vi "VibSystem2Signals.vi"(8 "sampling info":cluster{"Fs":dbl, "#s":dbl}={"Fs"=10000.0, "#s"=10000.0} {"Fs" format="%.2p"}, 10 "Frequency":dbl, 11 "Constant Amplitudes?":bool) -> (3 "Signals":waveform(dbl)[](array[waveform]))   [LabVIEW 2017]
uses:
  <vilib>/measure/NI_MABase.lvlib
panel:
  out "Waveform Graph":waveform(dbl)[](graph)
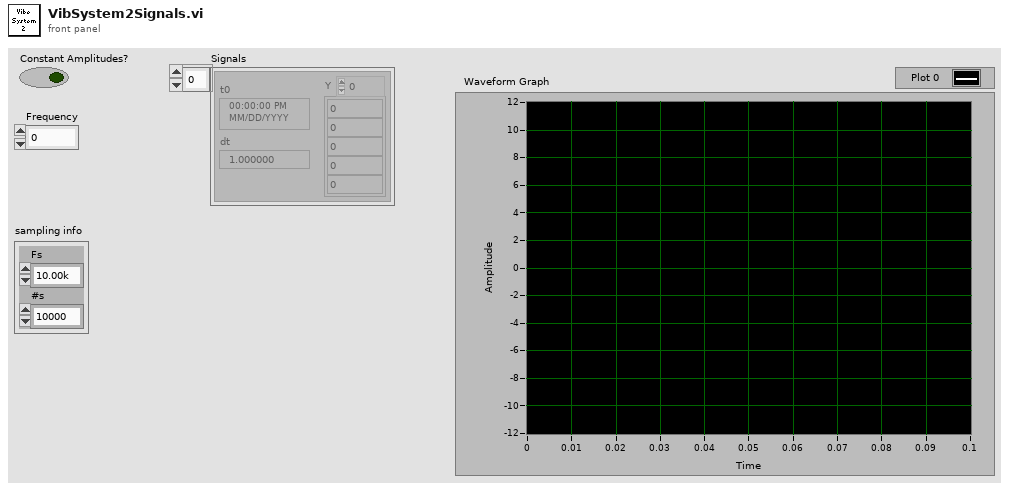
[diagram p1: front panel]
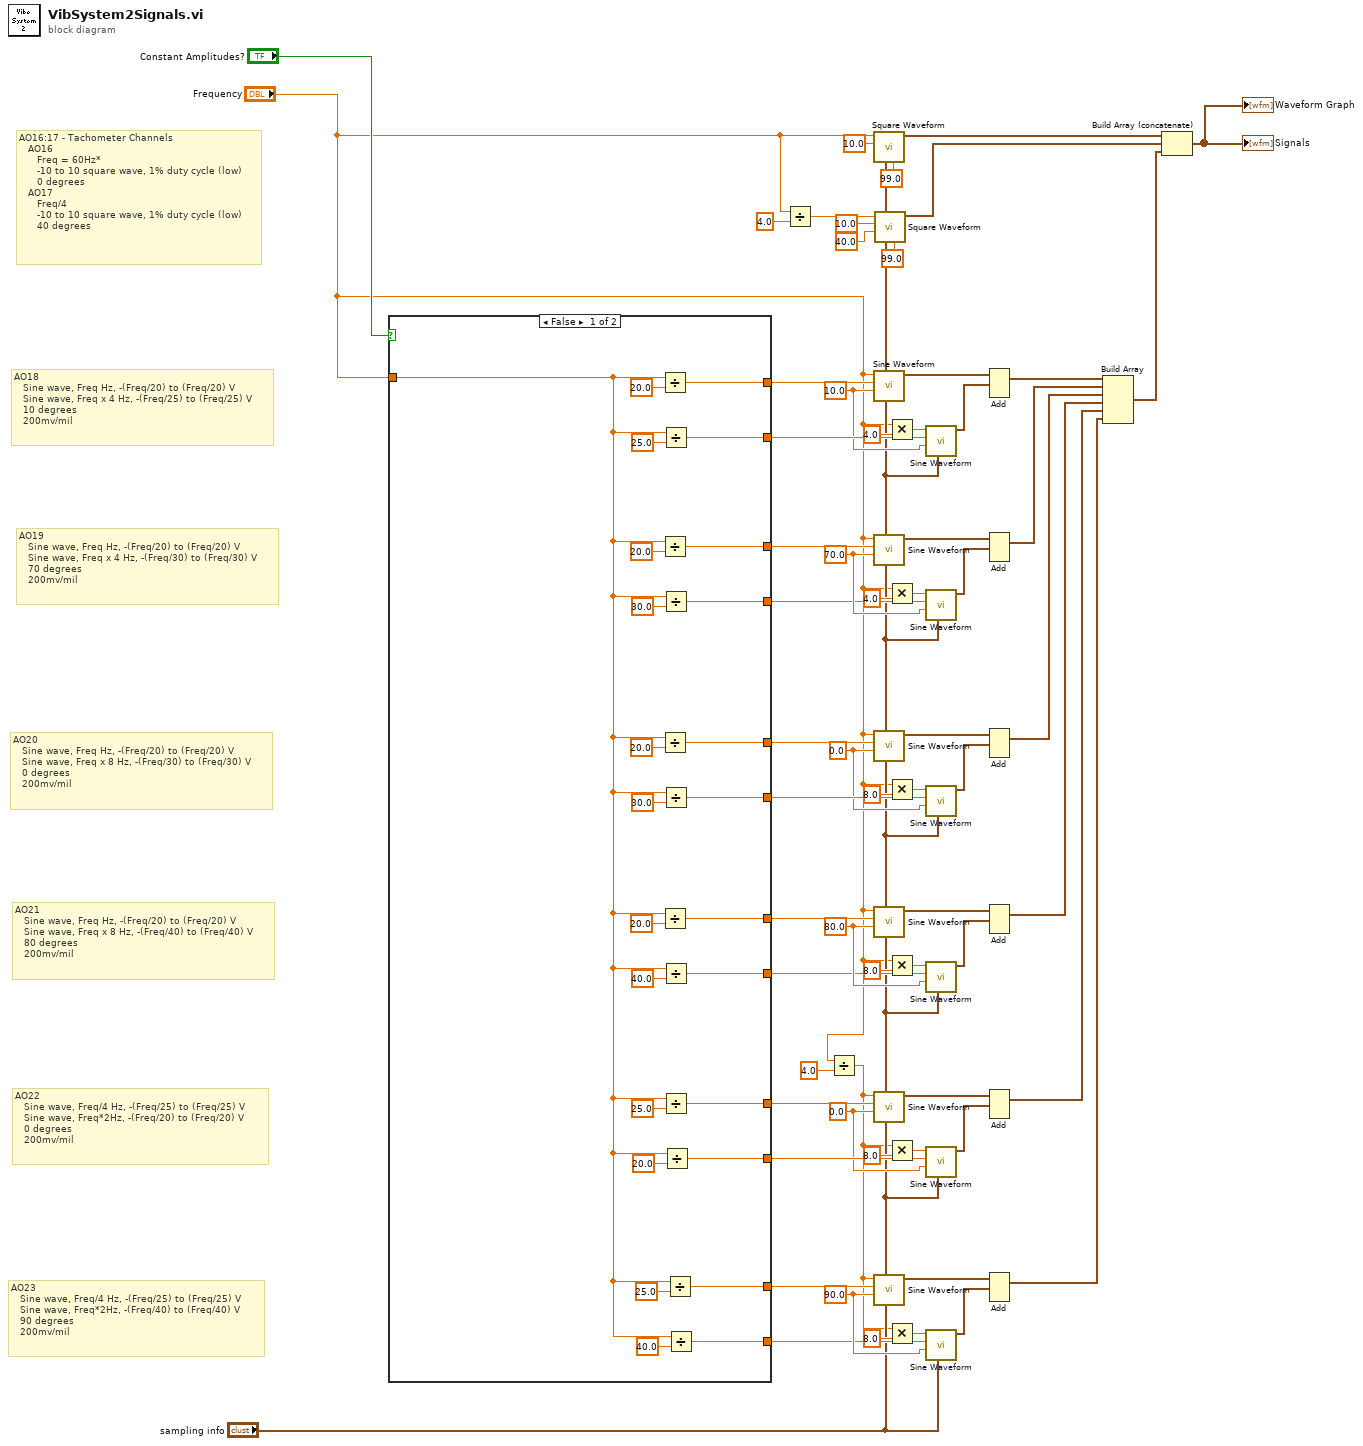
[diagram p0: block diagram]
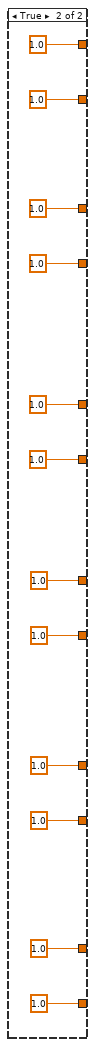
[diagram p2: hidden frame]
diagram:
  w9 = 90.0 ("phase")
  w18 = 0.0 ("phase")
  w24 = 80.0 ("phase")
  w34 = 0.0 ("phase")
  w40 = 70.0 ("phase")
  w60 = 10.0 ("phase")
  # "AO23\n   Sine wave, Freq/4 Hz, -(Freq/25) to (Freq/25) V\n   Sine wave, Freq*2Hz, -(Freq/40) to (Freq/40) V\n   90 degrees\n   200mv/mil"
  # "AO22\n   Sine wave, Freq/4 Hz, -(Freq/25) to (Freq/25) V\n   Sine wave, Freq*2Hz, -(Freq/20) to (Freq/20) V\n   0 degrees\n   200mv/mil"
  # "AO21\n   Sine wave, Freq Hz, -(Freq/20) to (Freq/20) V\n   Sine wave, Freq x 8 Hz, -(Freq/40) to (Freq/40) V\n   80 degrees\n   200mv/mil"
  # "AO19\n   Sine wave, Freq Hz, -(Freq/20) to (Freq/20) V\n   Sine wave, Freq x 4 Hz, -(Freq/30) to (Freq/30) V\n   70 degrees\n   200mv/mil"
  # "AO20\n   Sine wave, Freq Hz, -(Freq/20) to (Freq/20) V\n   Sine wave, Freq x 8 Hz, -(Freq/30) to (Freq/30) V\n   0 degrees\n   200mv/mil"
  # "AO18\n   Sine wave, Freq Hz, -(Freq/20) to (Freq/20) V\n   Sine wave, Freq x 4 Hz, -(Freq/25) to (Freq/25) V\n   10 degrees\n   200mv/mil"
  # "AO16:17 - Tachometer Channels\n   AO16\n      Freq = 60Hz*\n      -10 to 10 square wave, 1% duty cycle (low)\n      0 degrees\n   AO17\n      Freq/4\n      -10 to 10 square wave, 1% duty cycle (low)\n      40 degrees"
  n1 = case shown="False" "Constant Amplitudes?" {
    tunnel: [w87 1.0] -> w62
    tunnel: [w86 1.0] -> w63
    tunnel: "Frequency" -> [w69 _]
    tunnel: [w84 1.0] -> w39
    tunnel: [w85 1.0] -> w38
    tunnel: [w79 1.0] -> w35
    tunnel: [w78 1.0] -> w36
    tunnel: [w76 1.0] -> w23
    tunnel: [w77 1.0] -> w22
    tunnel: [w68 1.0] -> w19
    tunnel: [w67 1.0] -> w20
    tunnel: [w66 1.0] -> w8
    tunnel: [w65 1.0] -> w7
    frame False {
      n2 = Divide(x=w69, y=20.0) -> (x/y=w87:dbl)
      n3 = Divide(x=w69, y=20.0) -> (x/y=w84:dbl)
      n4 = Divide(x=w69, y=20.0) -> (x/y=w79:dbl)
      n5 = Divide(x=w69, y=20.0) -> (x/y=w76:dbl)
      n6 = Divide(x=w69, y=25.0) -> (x/y=w86:dbl)
      n7 = Divide(x=w69, y=30.0) -> (x/y=w85:dbl)
      n8 = Divide(x=w69, y=30.0) -> (x/y=w78:dbl)
      n9 = Divide(x=w69, y=40.0) -> (x/y=w77:dbl)
      n10 = Divide(x=w69, y=25.0) -> (x/y=w68:dbl)
      n11 = Divide(x=w69, y=20.0) -> (x/y=w67:dbl)
      n12 = Divide(x=w69, y=25.0) -> (x/y=w66:dbl)
      n13 = Divide(x=w69, y=40.0) -> (x/y=w65:dbl)
    }
    frame True {
    }
  }
  n14 = Divide(x="Frequency", y=4.0) -> (x/y=w47:dbl)
  n15 = Divide(x="Frequency", y=4.0) -> (x/y=w1:dbl)
  n16 = call <vilib>:"Square Waveform.vi"("duty cycle (%)"=99.0, "sampling info"="sampling info", "amplitude"=10.0, "frequency"="Frequency") -> ("signal out"=w55:waveform(dbl))  [unwired: 6 in, 1 out]
  n17 = call <vilib>:"Sine Waveform.vi"("sampling info"="sampling info", "phase"=w60, "amplitude"=w62, "frequency"="Frequency") -> ("signal out"=w59:waveform(dbl))  [unwired: 6 in, 1 out]
  n18 = call <vilib>:"Sine Waveform.vi"("sampling info"="sampling info", "phase"=w40, "amplitude"=w39, "frequency"="Frequency") -> ("signal out"=w41:waveform(dbl))  [unwired: 6 in, 1 out]
  n19 = call <vilib>:"Sine Waveform.vi"("sampling info"="sampling info", "phase"=w34, "amplitude"=w35, "frequency"="Frequency") -> ("signal out"=w33:waveform(dbl))  [unwired: 6 in, 1 out]
  n20 = call <vilib>:"Sine Waveform.vi"("sampling info"="sampling info", "phase"=w24, "amplitude"=w23, "frequency"="Frequency") -> ("signal out"=w25:waveform(dbl))  [unwired: 6 in, 1 out]
  n21 = call <vilib>:"Sine Waveform.vi"("sampling info"="sampling info", "phase"=w18, "amplitude"=w19, "frequency"=w1) -> ("signal out"=w17:waveform(dbl))  [unwired: 6 in, 1 out]
  n22 = call <vilib>:"Sine Waveform.vi"("sampling info"="sampling info", "phase"=w9, "amplitude"=w8, "frequency"=w1) -> ("signal out"=w10:waveform(dbl))  [unwired: 6 in, 1 out]
  n23 = call <vilib>:"Square Waveform.vi"("duty cycle (%)"=99.0, "sampling info"="sampling info", "phase"=40.0, "amplitude"=10.0, "frequency"=w47) -> ("signal out"=w48:waveform(dbl))  [unwired: 5 in, 1 out]
  n24 = Multiply(x="Frequency", y=4.0) -> (x*y=w56:dbl)
  n25 = Multiply(x="Frequency", y=4.0) -> (x*y=w44:dbl)
  n26 = Multiply(x="Frequency", y=8.0) -> (x*y=w30:dbl)
  n27 = Multiply(x="Frequency", y=8.0) -> (x*y=w28:dbl)
  n28 = Multiply(x=w1, y=8.0) -> (x*y=w14:dbl)
  n29 = Multiply(x=w1, y=8.0) -> (x*y=w13:dbl)
  n30 = call <vilib>:"Sine Waveform.vi"("sampling info"="sampling info", "phase"=w60, "amplitude"=w63, "frequency"=w56) -> ("signal out"=w58:waveform(dbl))  [unwired: 6 in, 1 out]
  n31 = call <vilib>:"Sine Waveform.vi"("sampling info"="sampling info", "phase"=w40, "amplitude"=w38, "frequency"=w44) -> ("signal out"=w42:waveform(dbl))  [unwired: 6 in, 1 out]
  n32 = call <vilib>:"Sine Waveform.vi"("sampling info"="sampling info", "phase"=w34, "amplitude"=w36, "frequency"=w30) -> ("signal out"=w32:waveform(dbl))  [unwired: 6 in, 1 out]
  n33 = call <vilib>:"Sine Waveform.vi"("sampling info"="sampling info", "phase"=w24, "amplitude"=w22, "frequency"=w28) -> ("signal out"=w26:waveform(dbl))  [unwired: 6 in, 1 out]
  n34 = call <vilib>:"Sine Waveform.vi"("sampling info"="sampling info", "phase"=w18, "amplitude"=w20, "frequency"=w14) -> ("signal out"=w16:waveform(dbl))  [unwired: 6 in, 1 out]
  n35 = call <vilib>:"Sine Waveform.vi"("sampling info"="sampling info", "phase"=w9, "amplitude"=w7, "frequency"=w13) -> ("signal out"=w11:waveform(dbl))  [unwired: 6 in, 1 out]
  n36 = Add(1:w58, 2:w59) -> (0:w64:waveform(dbl))  [unwired: 1 in, 1 out]
  n37 = Add(1:w42, 2:w41) -> (0:w37:waveform(dbl))  [unwired: 1 in, 1 out]
  n38 = Add(1:w32, 2:w33) -> (0:w29:waveform(dbl))  [unwired: 1 in, 1 out]
  n39 = Add(1:w26, 2:w25) -> (0:w21:waveform(dbl))  [unwired: 1 in, 1 out]
  n40 = Add(1:w16, 2:w17) -> (0:w5:waveform(dbl))  [unwired: 1 in, 1 out]
  n41 = Add(1:w11, 2:w10) -> (0:w4:waveform(dbl))  [unwired: 1 in, 1 out]
  n42 = Build Array(w64, w37, w29, w21, w5, w4) -> (w45:waveform(dbl)[])
  n43 = Build Array (concatenate)(w55, w48, w45) -> (→"Signals" →"Waveform Graph":waveform(dbl)[])
